vi "Test Execute SQL Query (double).vi"(8 "error in (no error)":errorcluster, 10 "query":string="SELECT * from employees;", 11 "database in":path=path "C:/labview/sqlite_dbManager/test database/chinook.db") -> (0 "error out":errorcluster, 1 "Query Result":dbl[][](array[numeric]), 2 "nonzero result?":bool)   [LabVIEW 2020, in "sqlite3.lvlib"]
uses:
  sqlite3.lvlib
panel:
  in  "desired return type":dbl
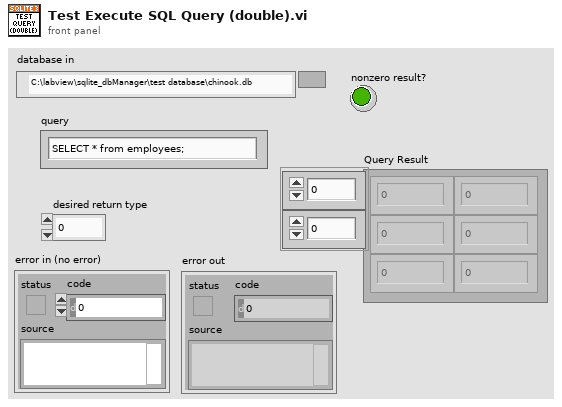
[diagram p1: front panel]
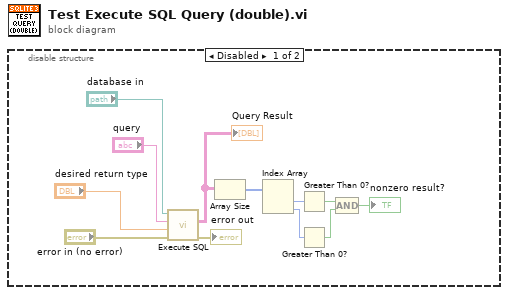
[diagram p0: block diagram]
diagram:
  n1 = disable-structure shown="Disabled" {
    frame Disabled {
      n2 = call "Execute SQL.vi"("error in (no error)"="error in (no error)", "[disabled] return type (string)"="desired return type", "sql (string)"="query", "database in"="database in") -> ("error out"=→"error out":errorcluster, "Query Result"=w7:string[][])  [unwired: 6 in]
      "Query Result" <- w7
      n3 = Array Size(array=w7) -> (size(s)=w6:i32[])
      n4 = Index Array(array=w6) -> (element #1=w5:i32, element #2=w4:i32)  [unwired: 2 in]
      n5 = Greater Than 0?(x=w5) -> (x > 0?=w3:bool)
      n6 = Greater Than 0?(x=w4) -> (x > 0?=w2:bool)
      n7 = Compound Arithmetic op=AND(w3, w2) -> (→"nonzero result?":bool)
    }
    frame Enabled {
    }
  }
